vi "Kernel_Convolution.vi"() -> ()   [LabVIEW 2017]
uses:
  <vilib>/vision/NI_Vision_Development_Module.lvlib
panel:
  out "Numeric 2":i32
  out "Numeric":i32
  out "Image 2":T1(plugin-control)
  out "error out":errorcluster
  out "Image":T1(plugin-control)
  out "Image File Selected":string
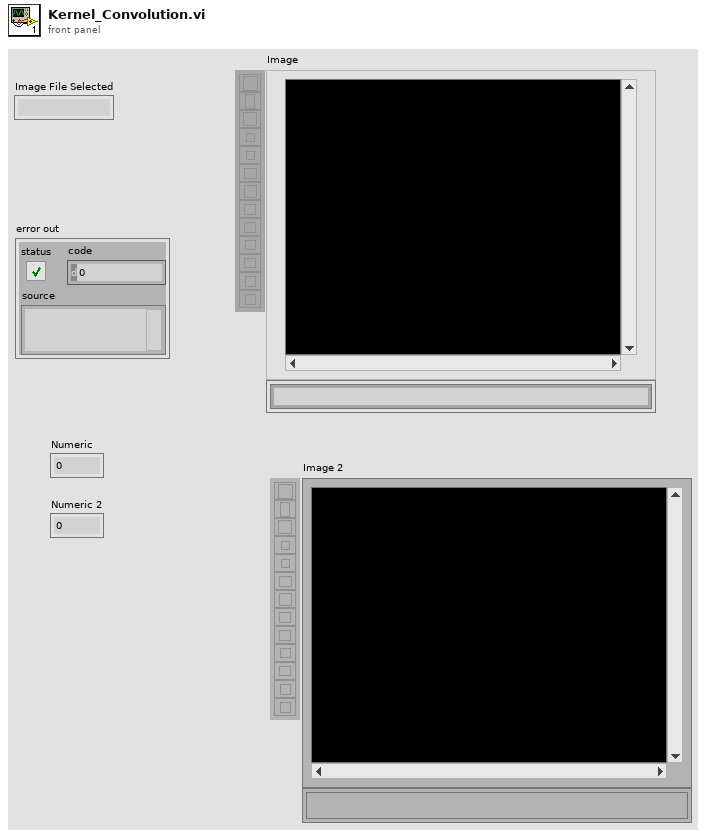
[diagram p1: front panel]
types:
  T1 = typedef "IMAQ Image.ctl" = refnum<image>
  T2 = typedef "Image Type" = u32
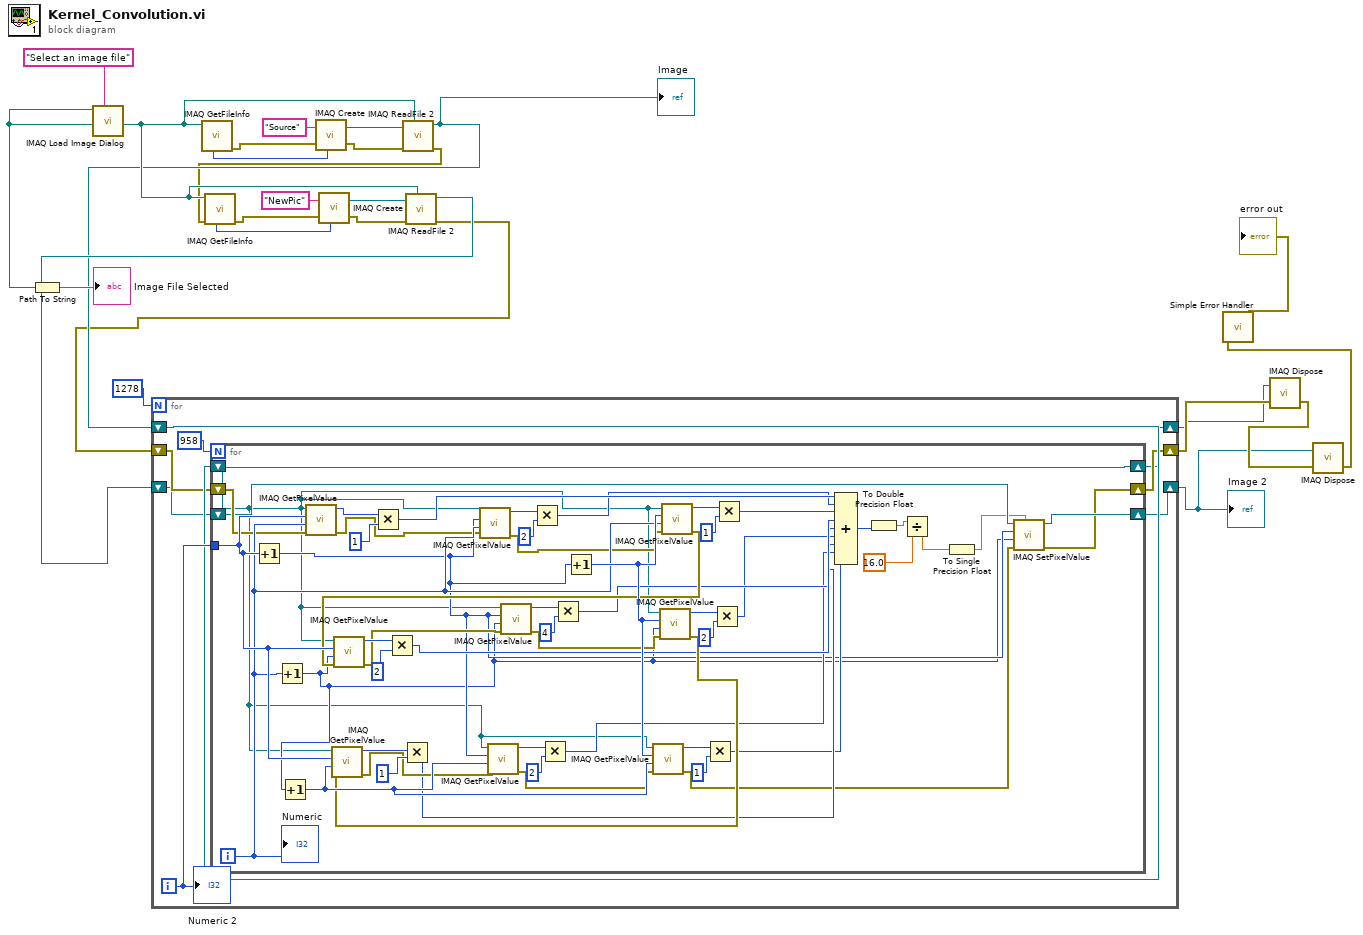
[diagram p0: block diagram]
diagram:
  n1 = call "IMAQ Load Image Dialog"("Prompt"="Select an image file") -> ("Path"=w11:path)  [unwired: 8 in, 2 out]
  n2 = Path To String(path=w11) -> (string=→"Image File Selected":string)
  n3 = call "IMAQ GetFileInfo"("File Path"=w11) -> ("error out"=w20:errorcluster, "Image Type"=w19:T2)  [unwired: 4 in, 5 out]
  n4 = call "IMAQ Create"("Image Name"="Source", "Image Type"=w19, "error in (no error)"=w20) -> ("New Image"=w17:T1, "error out"=w22:errorcluster)  [unwired: 2 in]
  n5 = call "IMAQ ReadFile 2"("File Path"=w11, "error in (no error)"=w22, "Image"=w17) -> ("error out"=w7:errorcluster, "Image Out"=w8:T1)  [unwired: 4 in, 3 out]
  "Image" <- w8
  n6 = call "IMAQ GetFileInfo"("error in (no error)"=w7, "File Path"=w11) -> ("error out"=w14:errorcluster, "Image Type"=w13:T2)  [unwired: 3 in, 5 out]
  n7 = call "IMAQ Create"("Image Name"="NewPic", "Image Type"=w13, "error in (no error)"=w14) -> ("New Image"=w12:T1, "error out"=w16:errorcluster)  [unwired: 2 in]
  n8 = call "IMAQ ReadFile 2"("File Path"=w11, "error in (no error)"=w16, "Image"=w12) -> ("error out"=w6:errorcluster, "Image Out"=w9:T1)  [unwired: 4 in, 3 out]
  n9 = for {
    N: 1278 -> [_]
    shift-right: [w27] -> w1
    shift-left: w9 -> [w28]
    shift-right: [w26] -> w5
    shift-left: w6 -> [w29]
    shift-right: [w25] -> w2
    shift-left: w8 -> [w30]
    i -> [w31]
    n10 = for {
      N: 958 -> [_]
      tunnel: w31 -> [w66]
      shift-right: [w35] -> w27
      shift-left: w28 -> [w41]
      shift-right: [w34] -> w26
      shift-left: w29 -> [w62]
      shift-right: [w33] -> w25
      shift-left: w30 -> [w33]
      i -> [w64]
      n11 = Increment(x=w66) -> (x+1=w37:i32)
      n12 = Increment(x=w64) -> (x+1=w36:i32)
      n13 = Increment(x=w36) -> (x+1=w63:i32)
      n14 = call "IMAQ GetPixelValue"("Image"=w33, "X Coordinate"=w66, "Y Coordinate"=w64, "error in (no error)"=w62) -> ("Pixel Value (U8)"=w84:u8, "error out"=w61:errorcluster)  [unwired: 2 in, 3 out]
      n15 = Multiply(x=w84, y=u8 1) -> (x*y=w53:u8)
      n16 = call "IMAQ GetPixelValue"("Image"=w33, "X Coordinate"=w37, "Y Coordinate"=w64, "error in (no error)"=w61) -> ("Pixel Value (U8)"=w78:u8, "error out"=w60:errorcluster)  [unwired: 2 in, 3 out]
      n17 = Multiply(x=w78, y=u8 2) -> (x*y=w52:u8)
      n18 = Increment(x=w37) -> (x+1=w65:i32)
      n19 = call "IMAQ GetPixelValue"("Image"=w33, "X Coordinate"=w65, "Y Coordinate"=w64, "error in (no error)"=w60) -> ("Pixel Value (U8)"=w72:u8, "error out"=w59:errorcluster)  [unwired: 2 in, 3 out]
      n20 = call "IMAQ GetPixelValue"("Image"=w33, "X Coordinate"=w66, "Y Coordinate"=w36, "error in (no error)"=w59) -> ("Pixel Value (U8)"=w82:u8, "error out"=w58:errorcluster)  [unwired: 2 in, 3 out]
      n21 = Multiply(x=w82, y=u8 2) -> (x*y=w50:u8)
      n22 = call "IMAQ GetPixelValue"("Image"=w33, "X Coordinate"=w37, "Y Coordinate"=w36, "error in (no error)"=w58) -> ("Pixel Value (U8)"=w76:u8, "error out"=w57:errorcluster)  [unwired: 2 in, 3 out]
      n23 = Multiply(x=w76, y=u8 4) -> (x*y=w49:u8)
      n24 = call "IMAQ GetPixelValue"("Image"=w33, "X Coordinate"=w65, "Y Coordinate"=w36, "error in (no error)"=w57) -> ("Pixel Value (U8)"=w70:u8, "error out"=w56:errorcluster)  [unwired: 2 in, 3 out]
      n25 = call "IMAQ GetPixelValue"("Image"=w33, "X Coordinate"=w66, "Y Coordinate"=w63, "error in (no error)"=w56) -> ("Pixel Value (U8)"=w80:u8, "error out"=w55:errorcluster)  [unwired: 2 in, 3 out]
      n26 = Multiply(x=w80, y=u8 1) -> (x*y=w47:u8)
      n27 = call "IMAQ GetPixelValue"("Image"=w33, "X Coordinate"=w37, "Y Coordinate"=w63, "error in (no error)"=w55) -> ("Pixel Value (U8)"=w74:u8, "error out"=w54:errorcluster)  [unwired: 2 in, 3 out]
      n28 = Multiply(x=w74, y=u8 2) -> (x*y=w46:u8)
      n29 = call "IMAQ GetPixelValue"("Image"=w33, "X Coordinate"=w65, "Y Coordinate"=w63, "error in (no error)"=w54) -> ("Pixel Value (U8)"=w68:u8, "error out"=w40:errorcluster)  [unwired: 2 in, 3 out]
      n30 = Multiply(x=w68, y=u8 1) -> (x*y=w45:u8)
      n31 = Multiply(x=w70, y=u8 2) -> (x*y=w48:u8)
      n32 = Multiply(x=w72, y=u8 1) -> (x*y=w51:u8)
      n33 = Compound Arithmetic op=ADD(w53, w52, w51, w50, w49, w48, w47, w46, w45) -> (w44:u8)
      n34 = To Double Precision Float(number=w44) -> (double precision float=w43:dbl)
      n35 = Divide(x=w43, y=16.0) -> (x/y=w39:dbl)
      n36 = To Single Precision Float(number=w39) -> (single precision float=w38:sgl)
      n37 = call "IMAQ SetPixelValue"("Pixel Value"=w38, "error in (no error)"=w40, "Y Coordinate"=w36, "X Coordinate"=w37, "Image"=w41) -> ("error out"=w34:errorcluster, "Image Out"=w35:T1)  [unwired: 5 in]
      "Numeric" <- w64
    }
    "Numeric 2" <- w31
  }
  "Image 2" <- w1
  n38 = call "IMAQ Dispose"("Image"=w2, "error in (no error)"=w5) -> ("error out"=w4:errorcluster)  [unwired: 4 in]
  n39 = call "IMAQ Dispose"("Image"=w1, "error in (no error)"=w4) -> ("error out"=w3:errorcluster)  [unwired: 4 in]
  n40 = call <vilib>:"Simple Error Handler.vi"("error in (no error)"=w3) -> ("error out"=→"error out":errorcluster)  [unwired: 4 in, 4 out]
